vi "SetChannelConfAll.vi"(8 "error in":errorcluster, 9 "ChannelProperty":T1, 10 "Channel Num":u32, 11 "CAN-NI":refnum<class "CAN-NI.lvclass">) -> (0 "error out":errorcluster, 3 "CAN-NI":refnum<class "CAN-NI.lvclass">)   [LabVIEW 2019, in "CAN-NI.lvlib" / "CAN-NI.lvclass"]
uses:
  CAN-NI.lvclass
  TypeDef/ChannelProperty.ctl
  CAN-Interface/TypeDef/Def-Termination.ctl
  CAN-Interface/TypeDef/Def-Transmit Mode.ctl
  CAN-Interface/TypeDef/Def-Protocol.ctl
  CAN-NI.lvclass/CAN-NI.ctl
  CAN-Interface/Class-Interface.lvclass
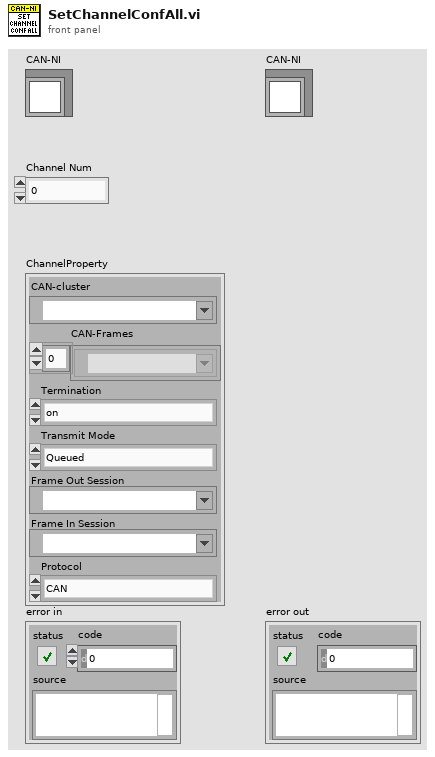
[diagram p1: front panel]
types:
  T1 = typedef "CAN-NI.lvlib/CAN-NI.lvclass/ChannelProperty.ctl" = cluster{"CAN-cluster":refnum<k21>, "CAN-Frames":refnum<k21>[], "Termination":T2, "Transmit Mode":T3, "Frame Out Session":refnum<k21>, "Frame In Session":refnum<k21>, "Protocol":T4}
  T2 = typedef "CAN-Interface.lvlib/Class-Interface.lvclass/Def-Termination.ctl" = enum8{"on", "off"}
  T3 = typedef "CAN-Interface.lvlib/Class-Interface.lvclass/Def-Transmit Mode.ctl" = enum16{"Queued", "Stream"}
  T4 = typedef "CAN-Interface.lvlib/Class-Interface.lvclass/Def-Protocol.ctl" = enum16{"CAN", "CAN FD"}
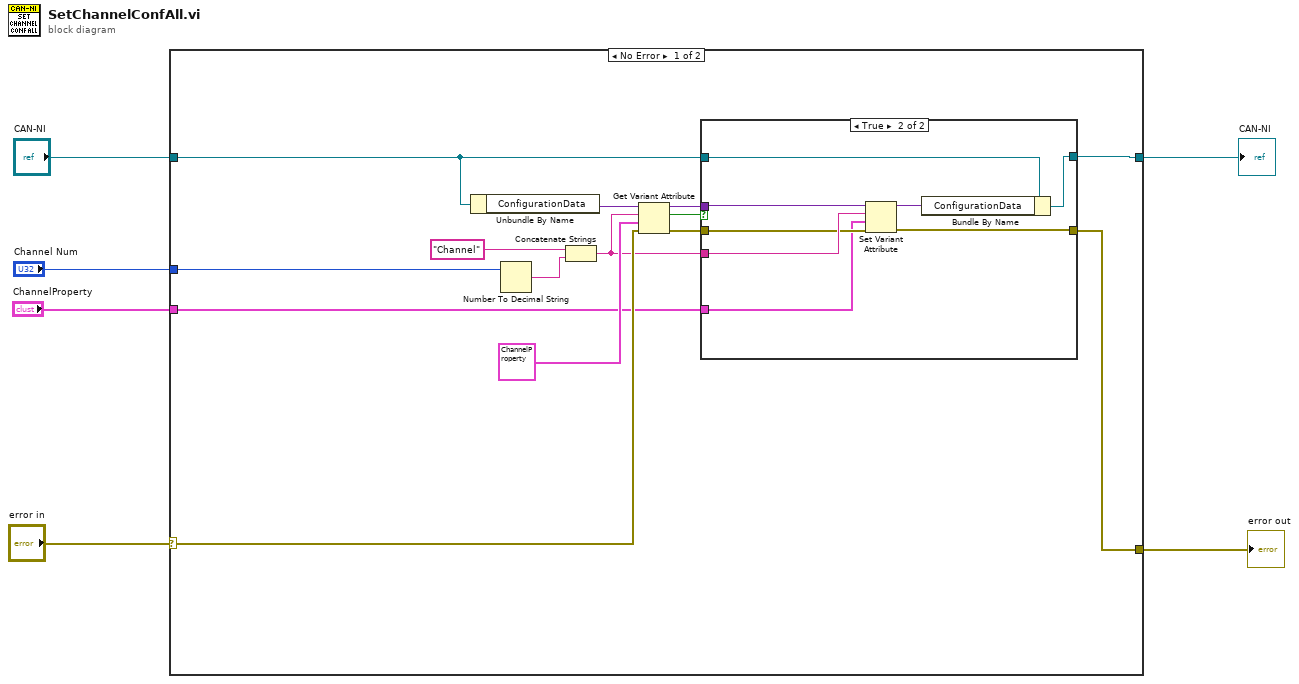
[diagram p0: block diagram]
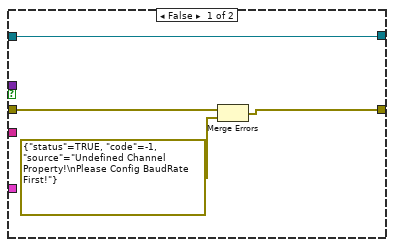
[diagram p2: hidden frame]
diagram:
  n1 = case shown="No Error" "error in" {
    selector: "error in" -> [w14 w34]
    tunnel: "CAN-NI" -> [w9 w33]
    tunnel: "Channel Num" -> [w18 _]
    tunnel: [w12 w34] -> w3
    tunnel: [w8 w33] -> w2
    tunnel: "ChannelProperty" -> [w7 _]
    frame No Error {
      n2 = Unbundle By Name(w9) -> ("ConfigurationData"=w17:variant)
      n3 = Number To Decimal String(number=w18) -> (decimal integer string=w20:string)  [unwired: 1 in]
      n4 = Concatenate Strings("Channel" ("string"), w20) -> (w10:string)
      n5 = Get Variant Attribute(Variant=w17, name=w10, default value (empty Variant)=T1 {"CAN-cluster"="", "CAN-Frames"=[], "Termination"=enum."on", "Transmit Mode"=enum."Queued", "Frame Out Session"="", "Frame In Session"="", "Protocol"=enum."CAN"} ("ChannelProperty"), error in=w14) -> (duplicate Variant=w11:variant, found=w15:bool, error out=w13:errorcluster)  [unwired: 1 out]
      n6 = case shown="True" w15 {
        tunnel: w13 -> [w24 w29]
        tunnel: [w22 w30] -> w12
        tunnel: w11 -> [_ w32]
        tunnel: w10 -> [_ w31]
        tunnel: w9 -> [w21 w28]
        tunnel: [w21 w26] -> w8
        tunnel: w7 -> [_ w25]
        frame False {
          n7 = Merge Errors(w24, errorcluster {"status"=TRUE, "code"=-1, "source"="Undefined Channel Property!\nPlease Config BaudRate First!"} ("error in (no error)")) -> (w22:errorcluster)
        }
        frame True {
          n8 = Set Variant Attribute(Variant=w32, name=w31, value=w25, error in=w29) -> (Variant out=w27:variant, error out=w30:errorcluster)  [unwired: 1 out]
          n9 = Bundle By Name(cluster=w28, "ConfigurationData"=w27) -> (w26:refnum<class "CAN-NI.lvclass">)
        }
      }
    }
    frame Error {
    }
  }
  "error out" <- w3
  "CAN-NI" <- w2
